vi "Begin.vi"(8 "error in":errorcluster) -> (0 "error out":errorcluster)   [LabVIEW 2016]
doc: "Called before other user functions, this VI can be used to open I/O refnums, load in file data, and do general program initialization. Notice that the <B>error out</B> terminal is simply used for data flow. Wiring it to other structures or subVIs ensures that this VI runs first."
uses:
  <vilib>/Rock Robotics/WPI/DriverStation/WPI_DriverStationRobotMode2.ctl
  <vilib>/Rock Robotics/WPI/Joystick/WPI_JoystickDeviceEnum.ctl
  <vilib>/Rock Robotics/SystemInterfaces/DIO/FPGA_DIOPWMChannel.ctl
  <vilib>/Rock Robotics/SystemInterfaces/DIO/FPGA_DIOChannel.ctl
  <vilib>/Rock Robotics/SystemInterfaces/i2clib/i2c_bus.ctl
  <vilib>/Rock Robotics/WPI/ThirdParty/CanMotor/TalonSRX/WPI_CANTalonSRX_APIControlMode.ctl
  <vilib>/Rock Robotics/WPI/ThirdParty/CanMotor/TalonSRX/WPI_CANTalonSRX_APIFeedbackSelect.ctl
  <vilib>/Rock Robotics/WPI/ThirdParty/CanMotor/TalonSRX/WPI_CANTalonSRX_BrakeOverride.ctl
  Robot Global Data.vi
  <vilib>/Rock Robotics/Network Tables/NT Write String Array.vi
  <vilib>/Rock Robotics/WPI/MotorControl/WPI_MotorControlOpen Talon.vi
  <vilib>/Rock Robotics/WPI/MotorControl/WPI_MotorControlOpen SPARK.vi
  <vilib>/Rock Robotics/WPI/RobotDrive/WPI_RobotDriveOpen4MotorWithExistingMotors.vi
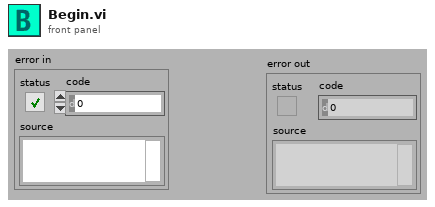
[diagram p1: front panel]
types:
  T1 = typedef "WPI_CANTalonSRX_BrakeOverride.ctl" = enum8{"No Override", "Override to Coast", "Override to Brake"}
  T2 = typedef "WPI_CANTalonSRX_APIControlMode.ctl" = enum8{"Percent VBus", "Speed", "Position", "Slave", "Unchanged / Invalid", "Voltage Compensation", "Current", "Motion Profile", "Motion Magic"}
  T3 = typedef "FPGA_DIOPWMChannel.ctl" = enum8{"PWM 0", "PWM 1", "PWM 2", "PWM 3", "PWM 4", "PWM 5", "PWM 6", "PWM 7", "PWM 8", "PWM 9", "PWM MXP 0", "PWM MXP 1", "PWM MXP 2", "PWM MXP 3", "PWM MXP 4", "PWM MXP 5", "PWM MXP 6", "PWM MXP 7", "PWM MXP 8", "PWM MXP 9", "Invalid"}
  T4 = typedef "WPI_CANTalonSRX_APIFeedbackSelect.ctl" = enum16{"Digital Quadrature Encoder", "Analog Potentiometer", "Analog Encoder", "Count on Quad-A (Rising-Edge)", "Count on Quad-A (Falling-Edge)", "CTR Magnetic Enc (Absolute)", "CTR Magnetic Enc (Relative)", "Pulse Width"}
  T5 = typedef "i2c_bus.ctl" = enum16{"I2C On-Board", "I2C MXP", "Invalid"}
  T6 = typedef "WPI_JoystickDeviceEnum.ctl" = enum16{"USB 0", "USB 1", "USB 2", "USB 3", "USB 4", "USB 5"}
  T7 = typedef "FPGA_DIOChannel.ctl" = enum8{"DIO 0", "DIO 1", "DIO 2", "DIO 3", "DIO 4", "DIO 5", "DIO 6", "DIO 7", "DIO 8", "DIO 9", "DIO MXP 0", "DIO MXP 1", "DIO MXP 2", "DIO MXP 3", "DIO MXP 4", "DIO MXP 5", "DIO MXP 6", "DIO MXP 7", "DIO MXP 8", "DIO MXP 9", "DIO MXP 10", "DIO MXP 11", "DIO MXP 12", "DIO MXP 13", "DIO MXP 14", "DIO MXP 15", "SPI Port CS1", "SPI Port CS2", "SPI Port CS3", "SPI Port MISO", "SPI Port MOSI", "Invalid"}
  T8 = typedef "WPI_DriverStationRobotMode2.ctl" = enum16{"Autonomous Disabled", "Autonomous Enabled", "Teleop Disabled", "Teleop Enabled", "Disconnected", "Finish", "Test Disabled", "Test Enabled", "Emergency Stopped"}
  T9 = typedef "WPI_MotorControlDeviceRef.ctl" = cluster{"DeviceStatus":errorcluster, "Type":T10, "PWM":cluster{"PWM Channel":T3, "DeadBand":T11}, "CAN":cluster{"Device Number":u8, "SetOutput VI Ref":variant, "GetOutput VI Ref":variant, "Enable VI Ref":variant, "Disable VI Ref":variant, "Data":variant}, "Invert":bool}
  T10 = typedef "WPI_MotorControlType.ctl" = enum16{"PWM", "CAN"}
  T11 = typedef "WPI_PWMDeadband.ctl" = cluster{"Name":string, "maxPositivePwm":i32, "minPositivePwm":i32, "centerPwm":i32, "maxNegativePwm":i32, "minNegativePwm":i32, "angularRange":u16}
  T12 = typedef "WPI_JoystickDevRef.ctl" = cluster{"Device":T6}
  T13 = typedef "WPI_I2CDevRef.ctl" = cluster{"DevStatus":errorcluster, "Device Address":u8, "Handle":i32, "I2C Bus":T5}
  T14 = typedef "WPI_DigitalInputDevRef.ctl" = cluster{"DevStatus":errorcluster, "DIO Channel":T7}
  T15 = typedef "WPI_RobotDriveDevRef.ctl" = cluster{"DevStatus":errorcluster, "Motors[]":T9[], "Square Inputs":bool, "Max Output":dbl}
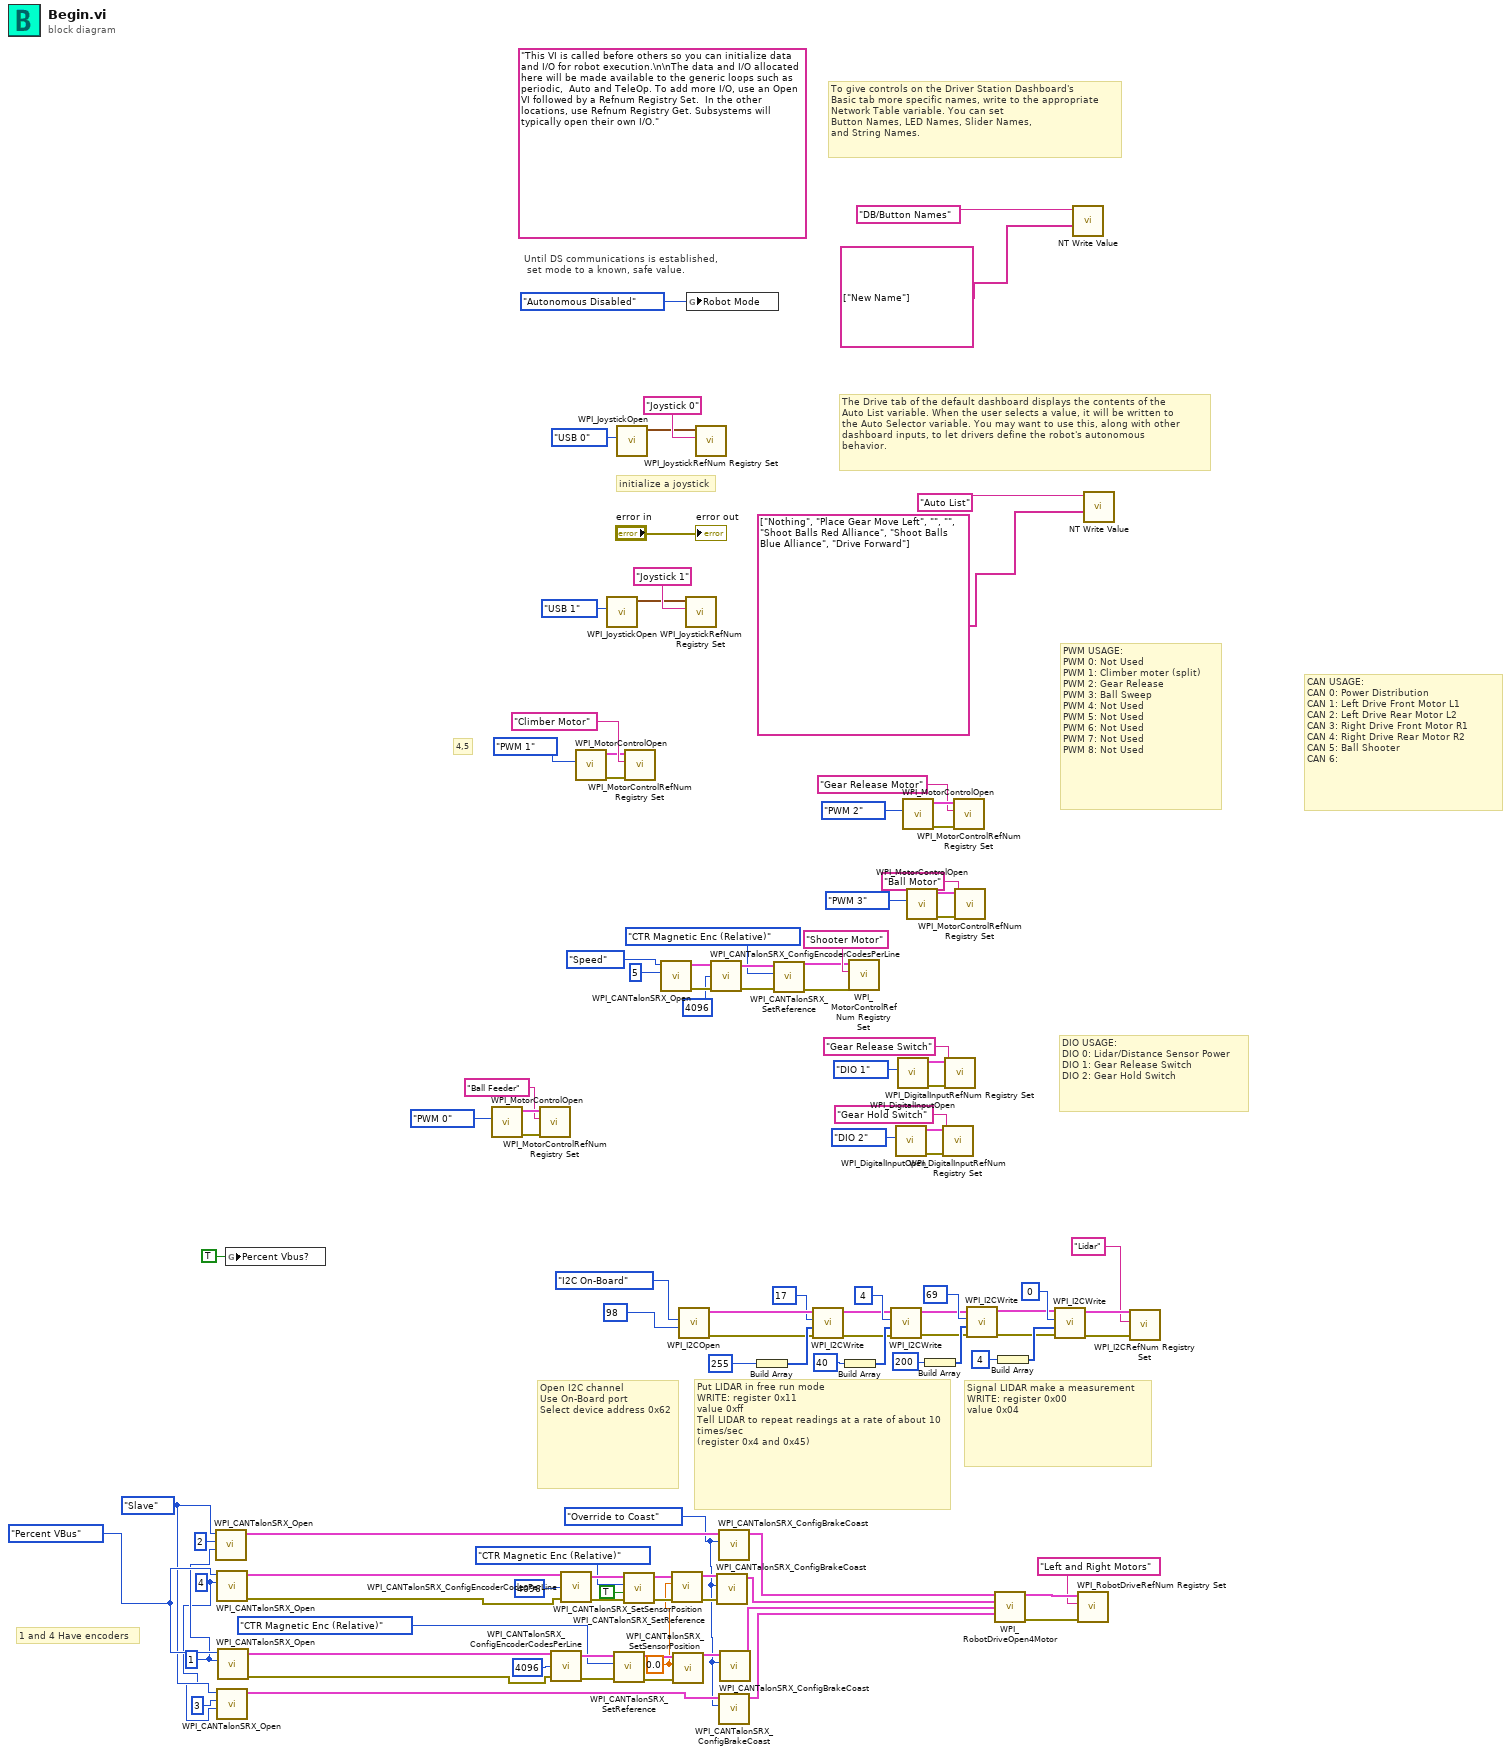
[diagram p0: block diagram]
diagram:
  w2 = WPI_CANTalonSRX_BrakeOverride."Override to Coast" ("Brake / Coast Mode")
  w16 = WPI_CANTalonSRX_APIControlMode."Slave" ("Control Mode")
  w22 = 0.0 ("New Sensor Position")
  w15 = u8 1 ("Device Number")
  w13 = u8 4 ("Device Number")
  w17 = WPI_CANTalonSRX_APIControlMode."Percent VBus" ("Control Mode")
  (unwired) "This VI is called before others so you can initialize data and I/O for robot execution.\n\nThe data and I/O allocated here will be made available to the generic loops such as periodic,  Auto and TeleOp. To add more I/O, use an Open VI followed by a Refnum Registry Set.  In the other locations, use Refnum Registry Get. Subsystems will typically open their own I/O."
  # "1 and 4 Have encoders"
  # "Signal LIDAR make a measurement\nWRITE: register 0x00\nvalue 0x04"
  # "Put LIDAR in free run mode\nWRITE: register 0x11\nvalue 0xff\nTell LIDAR to repeat readings at a rate of about 10 times/sec\n(register 0x4 and 0x45)"
  # "Open I2C channel\nUse On-Board port\nSelect device address 0x62"
  # "CAN USAGE:\nCAN 0: Power Distribution\nCAN 1: Left Drive Front Motor L1\nCAN 2: Left Drive Rear Motor L2\nCAN 3: Right Drive Front Motor R1\nCAN 4: Right Drive Rear Motor R2\nCAN 5: Ball Shooter\nCAN 6:"
  # "4,5"
  # "DIO USAGE:\nDIO 0: Lidar/Distance Sensor Power\nDIO 1: Gear Release Switch\nDIO 2: Gear Hold Switch"
  # "PWM USAGE:\nPWM 0: Not Used\nPWM 1: Climber moter (split) \nPWM 2: Gear Release\nPWM 3: Ball Sweep\nPWM 4: Not Used\nPWM 5: Not Used\nPWM 6: Not Used\nPWM 7: Not Used\nPWM 8: Not Used"
  # "The Drive tab of the default dashboard displays the contents of the\nAuto List variable. When the user selects a value, it will be written to\nthe Auto Selector variable. You may want to use this, along with other\ndashboard inputs, to let drivers define the robot's autonomous\nbehavior."
  # "To give controls on the Driver Station Dashboard's\nBasic tab more specific names, write to the appropriate\nNetwork Table variable. You can set\nButton Names, LED Names, Slider Names,\nand String Names."
  # "initialize a joystick"
  # "Until DS communications is established,\n set mode to a known, safe value."
  n1 = call <vilib>:"WPI_CANTalonSRX_Open.vi"("Master Device Number"=w15, "Device Number"=u8 2, "Control Mode"=w16) -> ("CAN Talon SRX Ref"=w3:T9)  [unwired: 7 in, 1 out]
  n2 = call <vilib>:"WPI_CANTalonSRX_Open.vi"("Device Number"=w13, "Control Mode"=w17) -> ("error out"=w33:errorcluster, "CAN Talon SRX Ref"=w34:T9)  [unwired: 8 in]
  n3 = call <vilib>:"WPI_CANTalonSRX_Open.vi"("Master Device Number"=w13, "Device Number"=u8 3, "Control Mode"=w16) -> ("CAN Talon SRX Ref"=w10:T9)  [unwired: 7 in, 1 out]
  n4 = call <vilib>:"WPI_CANTalonSRX_Open.vi"("Device Number"=w15, "Control Mode"=w17) -> ("error out"=w27:errorcluster, "CAN Talon SRX Ref"=w28:T9)  [unwired: 8 in]
  n5 = global write "Robot Global Data.vi" "Percent Vbus?"(TRUE ("Percent Vbus?")) -> ()
  n6 = call-poly <vilib>:"WPI_MotorControlOpen.vi"("PWM Channel"=FPGA_DIOPWMChannel."PWM 0") -> ("error out"=w20:errorcluster, "MotorControlDeviceRef"=w19:T9)  [unwired: 9 in]
  n7 = call <vilib>:"WPI_MotorControlRefNum Registry Set.vi"("error in (no error)"=w20, "refnum name"="Ball Feeder", "MotorControlDevRef"=w19) -> ()  [unwired: 7 in, 2 out]
  n8 = call <vilib>:"WPI_CANTalonSRX_ConfigEncoderCodesPerLine.vi"("CAN Talon SRX Ref"=w28, "Number Encoder Lines\n(Counts Per Rotation)"=u32 4096 ("Number Encoder Lines\n(Counts Per Rotation)"), "error in (no error)"=w27) -> ("CAN Talon SRX Ref"=w31:T9, "error out"=w30:errorcluster)  [unwired: 11 in]
  n9 = call <vilib>:"WPI_CANTalonSRX_ConfigEncoderCodesPerLine.vi"("CAN Talon SRX Ref"=w34, "Number Encoder Lines\n(Counts Per Rotation)"=u32 4096 ("Number Encoder Lines\n(Counts Per Rotation)"), "error in (no error)"=w33) -> ("CAN Talon SRX Ref"=w37:T9, "error out"=w36:errorcluster)  [unwired: 11 in]
  n10 = call-poly <vilib>:"WPI_MotorControlOpen.vi"("PWM Channel"=FPGA_DIOPWMChannel."PWM 1" ("Left Motor")) -> ("error out"=w95:errorcluster, "MotorControlDeviceRef"=w77:T9)  [unwired: 9 in]
  n11 = call <vilib>:"WPI_JoystickOpen.vi"("JoystickDevice"=WPI_JoystickDeviceEnum."USB 1") -> ("JoystickDevRef"=w81:T12)  [unwired: 10 in]
  n12 = call <vilib>:"WPI_CANTalonSRX_SetReference.vi"("error in (no error)"=w30, "Feedback Reference"=WPI_CANTalonSRX_APIFeedbackSelect."CTR Magnetic Enc (Relative)", "CAN Talon SRX Ref"=w31) -> ("error out"=w25:errorcluster, "CAN Talon SRX Ref"=w26:T9)  [unwired: 7 in]
  n13 = call <vilib>:"WPI_JoystickOpen.vi"("JoystickDevice"=WPI_JoystickDeviceEnum."USB 0") -> ("JoystickDevRef"=w108:T12)  [unwired: 10 in]
  n14 = call <vilib>:"WPI_CANTalonSRX_SetReference.vi"("error in (no error)"=w36, "Reverse Feedback Sensor"=TRUE, "Feedback Reference"=WPI_CANTalonSRX_APIFeedbackSelect."CTR Magnetic Enc (Relative)", "CAN Talon SRX Ref"=w37) -> ("error out"=w23:errorcluster, "CAN Talon SRX Ref"=w24:T9)  [unwired: 6 in]
  n15 = call <vilib>:"WPI_MotorControlRefNum Registry Set.vi"("error in (no error)"=w95, "refnum name"="Climber Motor", "MotorControlDevRef"=w77) -> ()  [unwired: 7 in, 2 out]
  n16 = call <vilib>:"WPI_CANTalonSRX_Open.vi"("Device Number"=u8 5, "Control Mode"=WPI_CANTalonSRX_APIControlMode."Speed") -> ("error out"=w49:errorcluster, "CAN Talon SRX Ref"=w50:T9)  [unwired: 8 in]
  n17 = call <vilib>:"WPI_CANTalonSRX_SetSensorPosition.vi"("error in (no error)"=w23, "New Sensor Position"=w22, "CAN Talon SRX Ref"=w24) -> ("error out"=w7:errorcluster, "CAN Talon SRX Ref"=w6:T9)  [unwired: 7 in]
  n18 = call <vilib>:"WPI_CANTalonSRX_SetSensorPosition.vi"("error in (no error)"=w25, "New Sensor Position"=w22, "CAN Talon SRX Ref"=w26) -> ("CAN Talon SRX Ref"=w8:T9)  [unwired: 7 in, 1 out]
  n19 = call <vilib>:"WPI_I2COpen.vi"("Device Address"=u8 98, "I2C Bus"=i2c_bus."I2C On-Board") -> ("error out"=w56:errorcluster, "I2CDevRef"=w74:T13)  [unwired: 8 in]
  n20 = call <vilib>:"WPI_JoystickRefNum Registry Set.vi"("refnum name"="Joystick 1", "JoystickDevRef"=w81) -> ()  [unwired: 8 in, 2 out]
  n21 = global write "Robot Global Data.vi" "Robot Mode"(WPI_DriverStationRobotMode2."Autonomous Disabled" ("Robot Mode")) -> ()
  n22 = call <vilib>:"WPI_JoystickRefNum Registry Set.vi"("refnum name"="Joystick 0", "JoystickDevRef"=w108) -> ()  [unwired: 8 in, 2 out]
  n23 = call <vilib>:"WPI_CANTalonSRX_ConfigEncoderCodesPerLine.vi"("CAN Talon SRX Ref"=w50, "Number Encoder Lines\n(Counts Per Rotation)"=u32 4096 ("Number Encoder Lines\n(Counts Per Rotation)"), "error in (no error)"=w49) -> ("CAN Talon SRX Ref"=w45:T9, "error out"=w44:errorcluster)  [unwired: 11 in]
  n24 = call <vilib>:"WPI_CANTalonSRX_ConfigBrakeCoast.vi"("error in (no error)"=w7, "Brake / Coast Mode"=w2, "CAN Talon SRX Ref"=w6) -> ("CAN Talon SRX Ref"=w5:T9)  [unwired: 7 in, 1 out]
  n25 = call <vilib>:"WPI_CANTalonSRX_ConfigBrakeCoast.vi"("Brake / Coast Mode"=w2, "CAN Talon SRX Ref"=w3) -> ("CAN Talon SRX Ref"=w4:T9)  [unwired: 8 in, 1 out]
  n26 = call <vilib>:"WPI_CANTalonSRX_ConfigBrakeCoast.vi"("Brake / Coast Mode"=w2, "CAN Talon SRX Ref"=w10) -> ("CAN Talon SRX Ref"=w11:T9)  [unwired: 8 in, 1 out]
  n27 = call <vilib>:"WPI_CANTalonSRX_ConfigBrakeCoast.vi"("Brake / Coast Mode"=w2, "CAN Talon SRX Ref"=w8) -> ("CAN Talon SRX Ref"=w9:T9)  [unwired: 8 in, 1 out]
  n28 = Build Array(u8 255 ("Device Address")) -> (w71:u8[])
  n29 = call <vilib>:"WPI_CANTalonSRX_SetReference.vi"("error in (no error)"=w44, "Feedback Reference"=WPI_CANTalonSRX_APIFeedbackSelect."CTR Magnetic Enc (Relative)", "CAN Talon SRX Ref"=w45) -> ("error out"=w47:errorcluster, "CAN Talon SRX Ref"=w46:T9)  [unwired: 7 in]
  n30 = call <vilib>:"WPI_I2CWrite.vi"("error in (no error)"=w56, "I2CDataToSend"=w71, "I2CRegister"=u8 17 ("Device Address"), "I2CDevRef"=w74) -> ("error out"=w57:errorcluster, "I2CDevRef"=w61:T13)  [unwired: 6 in]
  n31 = Build Array(u8 40 ("Device Address")) -> (w66:u8[])
  n32 = call <vilib>:"WPI_MotorControlRefNum Registry Set.vi"("error in (no error)"=w47, "refnum name"="Shooter Motor", "MotorControlDevRef"=w46) -> ()  [unwired: 7 in, 2 out]
  n33 = call <vilib>:"WPI_I2CWrite.vi"("error in (no error)"=w57, "I2CDataToSend"=w66, "I2CRegister"=u8 4 ("Device Address"), "I2CDevRef"=w61) -> ("error out"=w58:errorcluster, "I2CDevRef"=w60:T13)  [unwired: 6 in]
  n34 = call <vilib>:"WPI_DigitalInputOpen.vi"("DIO Channel"=FPGA_DIOChannel."DIO 2") -> ("error out"=w91:errorcluster, "DigitalInputDevRef"=w90:T14)  [unwired: 9 in]
  n35 = call <vilib>:"WPI_DigitalInputOpen.vi"("DIO Channel"=FPGA_DIOChannel."DIO 1") -> ("error out"=w87:errorcluster, "DigitalInputDevRef"=w86:T14)  [unwired: 9 in]
  n36 = call-poly <vilib>:"WPI_MotorControlOpen.vi"("PWM Channel"=FPGA_DIOPWMChannel."PWM 2") -> ("error out"=w99:errorcluster, "MotorControlDeviceRef"=w98:T9)  [unwired: 9 in]
  n37 = call-poly <vilib>:"WPI_MotorControlOpen.vi"("PWM Channel"=FPGA_DIOPWMChannel."PWM 3") -> ("error out"=w97:errorcluster, "MotorControlDeviceRef"=w96:T9)  [unwired: 9 in]
  n38 = Build Array(u8 200 ("Device Address")) -> (w63:u8[])
  n39 = call <vilib>:"WPI_DigitalInputRefNum Registry Set.vi"("error in (no error)"=w91, "refnum name"="Gear Hold Switch", "DigitalInputDevRef"=w90) -> ()  [unwired: 7 in, 2 out]
  n40 = call <vilib>:"WPI_DigitalInputRefNum Registry Set.vi"("error in (no error)"=w87, "refnum name"="Gear Release Switch", "DigitalInputDevRef"=w86) -> ()  [unwired: 7 in, 2 out]
  n41 = call <vilib>:"WPI_MotorControlRefNum Registry Set.vi"("error in (no error)"=w99, "refnum name"="Gear Release Motor", "MotorControlDevRef"=w98) -> ()  [unwired: 7 in, 2 out]
  n42 = call <vilib>:"WPI_MotorControlRefNum Registry Set.vi"("error in (no error)"=w97, "refnum name"="Ball Motor", "MotorControlDevRef"=w96) -> ()  [unwired: 7 in, 2 out]
  n43 = call <vilib>:"WPI_I2CWrite.vi"("error in (no error)"=w58, "I2CDataToSend"=w63, "I2CRegister"=u8 69 ("Device Address"), "I2CDevRef"=w60) -> ("error out"=w55:errorcluster, "I2CDevRef"=w59:T13)  [unwired: 6 in]
  n44 = call-poly <vilib>:"WPI_RobotDriveOpen4Motor.vi"("Rear Left Motor Dev Ref"=w4, "Rear Right Motor Dev Ref"=w5, "Front Left Motor Dev Ref"=w9, "Front Right Motor Dev Ref"=w11) -> ("RobotDriveDevRef"=w42:T15, "error out"=w40:errorcluster)  [unwired: 10 in]
  n45 = Build Array(u8 4 ("Device Address")) -> (w68:u8[])
  n46 = call <vilib>:"WPI_I2CWrite.vi"("error in (no error)"=w55, "I2CDataToSend"=w68, "I2CRegister"=u8 0 ("Device Address"), "I2CDevRef"=w59) -> ("error out"=w53:errorcluster, "I2CDevRef"=w54:T13)  [unwired: 6 in]
  n47 = call-poly <vilib>:"NT Write Value.vi"("String Array"=string[] ["New Name"], "Name"="DB/Button Names") -> ()  [unwired: 9 in, 1 out]
  n48 = call <vilib>:"WPI_RobotDriveRefNum Registry Set.vi"("error in (no error)"=w40, "refnum name"="Left and Right Motors", "RobotDriveDevRef"=w42) -> ()  [unwired: 1 in, 8 out]
  n49 = call-poly <vilib>:"NT Write Value.vi"("String Array"=string[] ["Nothing", "Place Gear Move Left", "", "", "Shoot Balls Red Alliance", "Shoot Balls Blue Alliance", "Drive Forward"], "Name"="Auto List") -> ()  [unwired: 9 in, 1 out]
  n50 = call <vilib>:"WPI_I2CRefNum Registry Set.vi"("error in (no error)"=w53, "refnum name"="Lidar", "I2CDevRef"=w54) -> ()  [unwired: 7 in, 2 out]
  "error out" <- "error in"
